vi "Fpga-Mac-Top.vi"(9 "RX_FIFO_DATA":refnum<k21>="TH-RX_FIFO_DATA", 10 "RX_PKT":refnum<k21>="TH-RX_NEW_PKT", 11 "TX_FIFO":refnum<k21>="HT-TX_FIFO") -> ()   [LabVIEW 2017]
uses:
  <instrlib>/_niInstr/Network/Ethernet/MAC/CLIP/v1/Resources.ctl
  TX-States.ctl
  <vilib>/Platform/TimedLoop/XDataNode/timing_clust.ctl
  <vilib>/Platform/TimedLoop/XDataNode/nitl_modes.ctl
  <vilib>/Platform/TimedLoop/XDataNode/wakeup.ctl
  <instrlib>/_niInstr/Network/Ethernet/MAC/Raw Stream/v1/niInstr Ethernet MAC Raw Stream v1.lvclass
  <instrlib>/_niInstr/Network/Ethernet/Utility/v1/FPGA/Network Data Stream.ctl
  <vilib>/rvi/Emulation/niFpgaSctlEmulationGetInTimedLoop.vi
  <vilib>/rvi/Emulation/niFpgaEmulationReportErrorSimple.vi
  <vilib>/rvi/Emulation/niFpgaGetClockAttributes.vi
  <vilib>/rvi/Emulation/niFpgaCriticalErrorInLSC.vi
  <vilib>/rvi/DataTransferAndStorage/Container/Common/niFpgaContainerExecOnDevCompGetState.vi
  <vilib>/rvi/Emulation/niFpgaEmulationIsFPGAContextNoSignature.vi
  <vilib>/rvi/errors/niFpgaSetErrorForExecOnDevCompSimple.vi
  <vilib>/rvi/eio/common/nirviEmuReportErrorAndStop.vi
  <vilib>/rvi/DataTransferAndStorage/Container/Common/niFpgaContainerGetUniqueNameForEmu.vi
  <vilib>/rvi/FIFO/Fifo_Resource/nirvififoEmulationSetSize.vi
  <vilib>/rvi/FIFO/Fifo_Resource/nirviFifoEmulationQueueMgr.vi
  <instcachedir>/0/nirviFifoEmulationQueueMgr_E5CAEC123FF24DC58D834DCA3CDAA9B5.lvgen/nirviFifoEmulationQueueMgr_E5CAEC123FF24DC58D834DCA3CDAA9B5_000.vi
  <vilib>/rvi/FIFO/Fifo_Resource/nirvififoEmulationDetermineInputValidOut.vi
  <vilib>/rvi/FIFO/Fifo_Resource/nirvififoEmulationCreateLock.vi
  <vilib>/rvi/Emulation/niFpgaProcessEmulError.vi
  <vilib>/rvi/FIFO/Fifo_Resource/nirvififoEmulationObtainLock.vi
  <vilib>/rvi/FIFO/Fifo_Resource/nirvififoEmulationReleaseLock.vi
  <vilib>/rvi/occurrence/nirviWaitOnOccurrenceBase.vi
  <vilib>/rvi/errors/nirviReportUnexpectedCaseInternalError.vi
  <vilib>/rvi/errors/nirviReportUnexpectedCaseInternalError (U32).vi
  <vilib>/Utility/error.llb/Clear Errors.vi
  <vilib>/rvi/interface/RandomDataEmulation/niFpgaRandomDataHandleErrors.vi
  <instrlib>/_niInstr/Network/Ethernet/MAC/Raw Stream/v1/Write Data Stream.vi
  <instrlib>/_niInstr/Network/Ethernet/MAC/Raw Stream/v1/Write End of Good Frame.vi
  <instrlib>/_niInstr/Network/Ethernet/MAC/Raw Stream/v1/Read End of Bad Frame.vi
  <instrlib>/_niInstr/Network/Ethernet/MAC/Raw Stream/v1/Read End of Good Frame.vi
  <instrlib>/_niInstr/Network/Ethernet/MAC/Raw Stream/v1/Read Data Stream.vi
  <vilib>/rvi/interface/RandomDataEmulation/nirviRandomDataAcquireLock.vi
  <vilib>/rvi/interface/RandomDataEmulation/nirviRandomDataQueueStore.vi
  <vilib>/rvi/interface/RandomDataEmulation/nirviRandomDataReleaseLock.vi
  <vilib>/rvi/interface/RandomDataEmulation/nirviFPGAContextMergeError.vi
  <vilib>/rvi/interface/RandomDataEmulation/nirviRandomDataCheckExitLoopConditions.vi
  <vilib>/express/rvi/timingcommon/nirviCommon.vi
  <instcachedir>/0/nirviFifoEmulationQueueMgr_E5CAEC123FF24DC58D834DCA3CDAA9B5.lvgen/nirviFifoEmulationQueueMgr_E5CAEC123FF24DC58D834DCA3CDAA9B5_007.vi
  <vilib>/rvi/eio/common/nirviEmuTemplateMethod_errors.vi
  <vilib>/Platform/TimedLoop/XDataNode/XDataNode.xnode
  <vilib>/rvi/DataTransferAndStorage/Container/XNode/niFpgaContainer.xnode
  <vilib>/rvi/FIFO/Fifo_Resource/niFpgaFifoEmulationRefIn.vi
  <vilib>/rvi/FIFO/Fifo_Resource/niFpgaFifoEmulationRefInMultiElement.vi
  <vilib>/eio/EIONode/EIONode.xnode
  <instrlib>/_niInstr/Network/Ethernet/MAC/CLIP/v1/niInstr Ethernet MAC - CLIP v1.lvclass
  <vilib>/Platform/TimedLoop/XDataNode/XDNodeRunTimeDep.lvlib
  <instrlib>/_niInstr/Network/Ethernet/Utility/v1/FPGA/niInstr Ethernet Utilities FPGA v1.lvlib
panel:
  out "mgtrefclks_locked":bool
  out "mgtrefclks_valid":bool
  out "posc_complete":bool
  out "sPort0_Power_Good":bool
  out "sPort1_Power_Good":bool
  out "signal_detect_Port0":bool
  out "signal_detect_Port1":bool
  out "aBlockLockPort0":bool
  out "aBlockLockPort1":bool
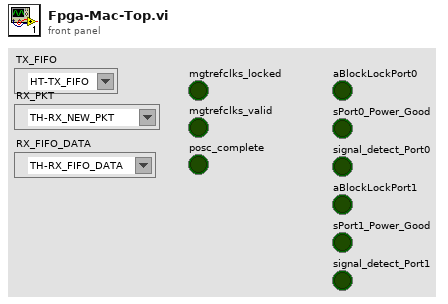
[diagram p1: front panel]
types:
  T1 = typedef "TX-States.ctl" = enum16{"Idle", "ReadSize", "WaitForData", "ReadData", "Reset", "InterFrameGap"}
  T2 = typedef "niInstr Ethernet MAC - CLIP v1.lvclass/Resources.ctl" = cluster{"RX":cluster{"TData":refnum<k21>, "TValid":refnum<k21>, "TKeep":refnum<k21>, "TLast":refnum<k21>, "TUser":refnum<k21>}, "TX":cluster{"TData":refnum<k21>, "TValid":refnum<k21>, "TKeep":refnum<k21>, "TLast":refnum<k21>, "TReady":refnum<k21>}, "Pause resources":cluster{"cPauseValuePort":refnum<k21>, "cPauseReqPort":refnum<k21>}, "MAC Clock":refnum<k21>}
  T3 = typedef "XDNodeRunTimeDep.lvlib/timing_clust.ctl" = cluster{"Expected End [f-1]":u64, "Actual End [f-1]":u64, "Finished Late? [f-1]":bool, "Expected End [i-1]":u64, "Actual End [i-1]":u64, "Finished Late? [i-1]":bool, "Expected Start [i]":u64, "Actual Start [i]":u64, "Expected Start [f]":u64, "Actual Start [f]":u64, "Source Name":string, "Structure Name":string, "Period":i64, "Deadline":i64, "Offset":i64, "Start":i64, "Priority":i32, "Timeout":i32, "Mode":T4, "Wakeup Reason":T5, "Error":errorcluster, "Source Type":string, "Secondary Source Type":string, "Global End Time":u64, "Global Start Time":u64, "Frame Duration":u64, "Iteration Duration":u64, "Assigned CPU":i32, "I/O Scan Engine Mode":u32}
  T4 = typedef "XDNodeRunTimeDep.lvlib/nitl_modes.ctl" = enum32{"No Change", "Process missed periods, maintain original phase", "Discard missed periods, maintain original phase", "Process missed periods, ignore original phase", "Discard missed periods, ignore original phase"}
  T5 = typedef "XDNodeRunTimeDep.lvlib/wakeup.ctl" = enum32{"Normal", "Aborted", "Asynchronous wakeup", "Timing source error", "Timed loop error", "Timeout"}
  T6 = cluster{"TotalBytes":u32, "TotalWords":u32, "Remainder":u32, "Counter":u32}
  T7 = typedef "niInstr Ethernet Utilities FPGA v1.lvlib/Network Data Stream.ctl" = cluster{"data":u8[], "data valid":bool, "byte enables":bool[]}
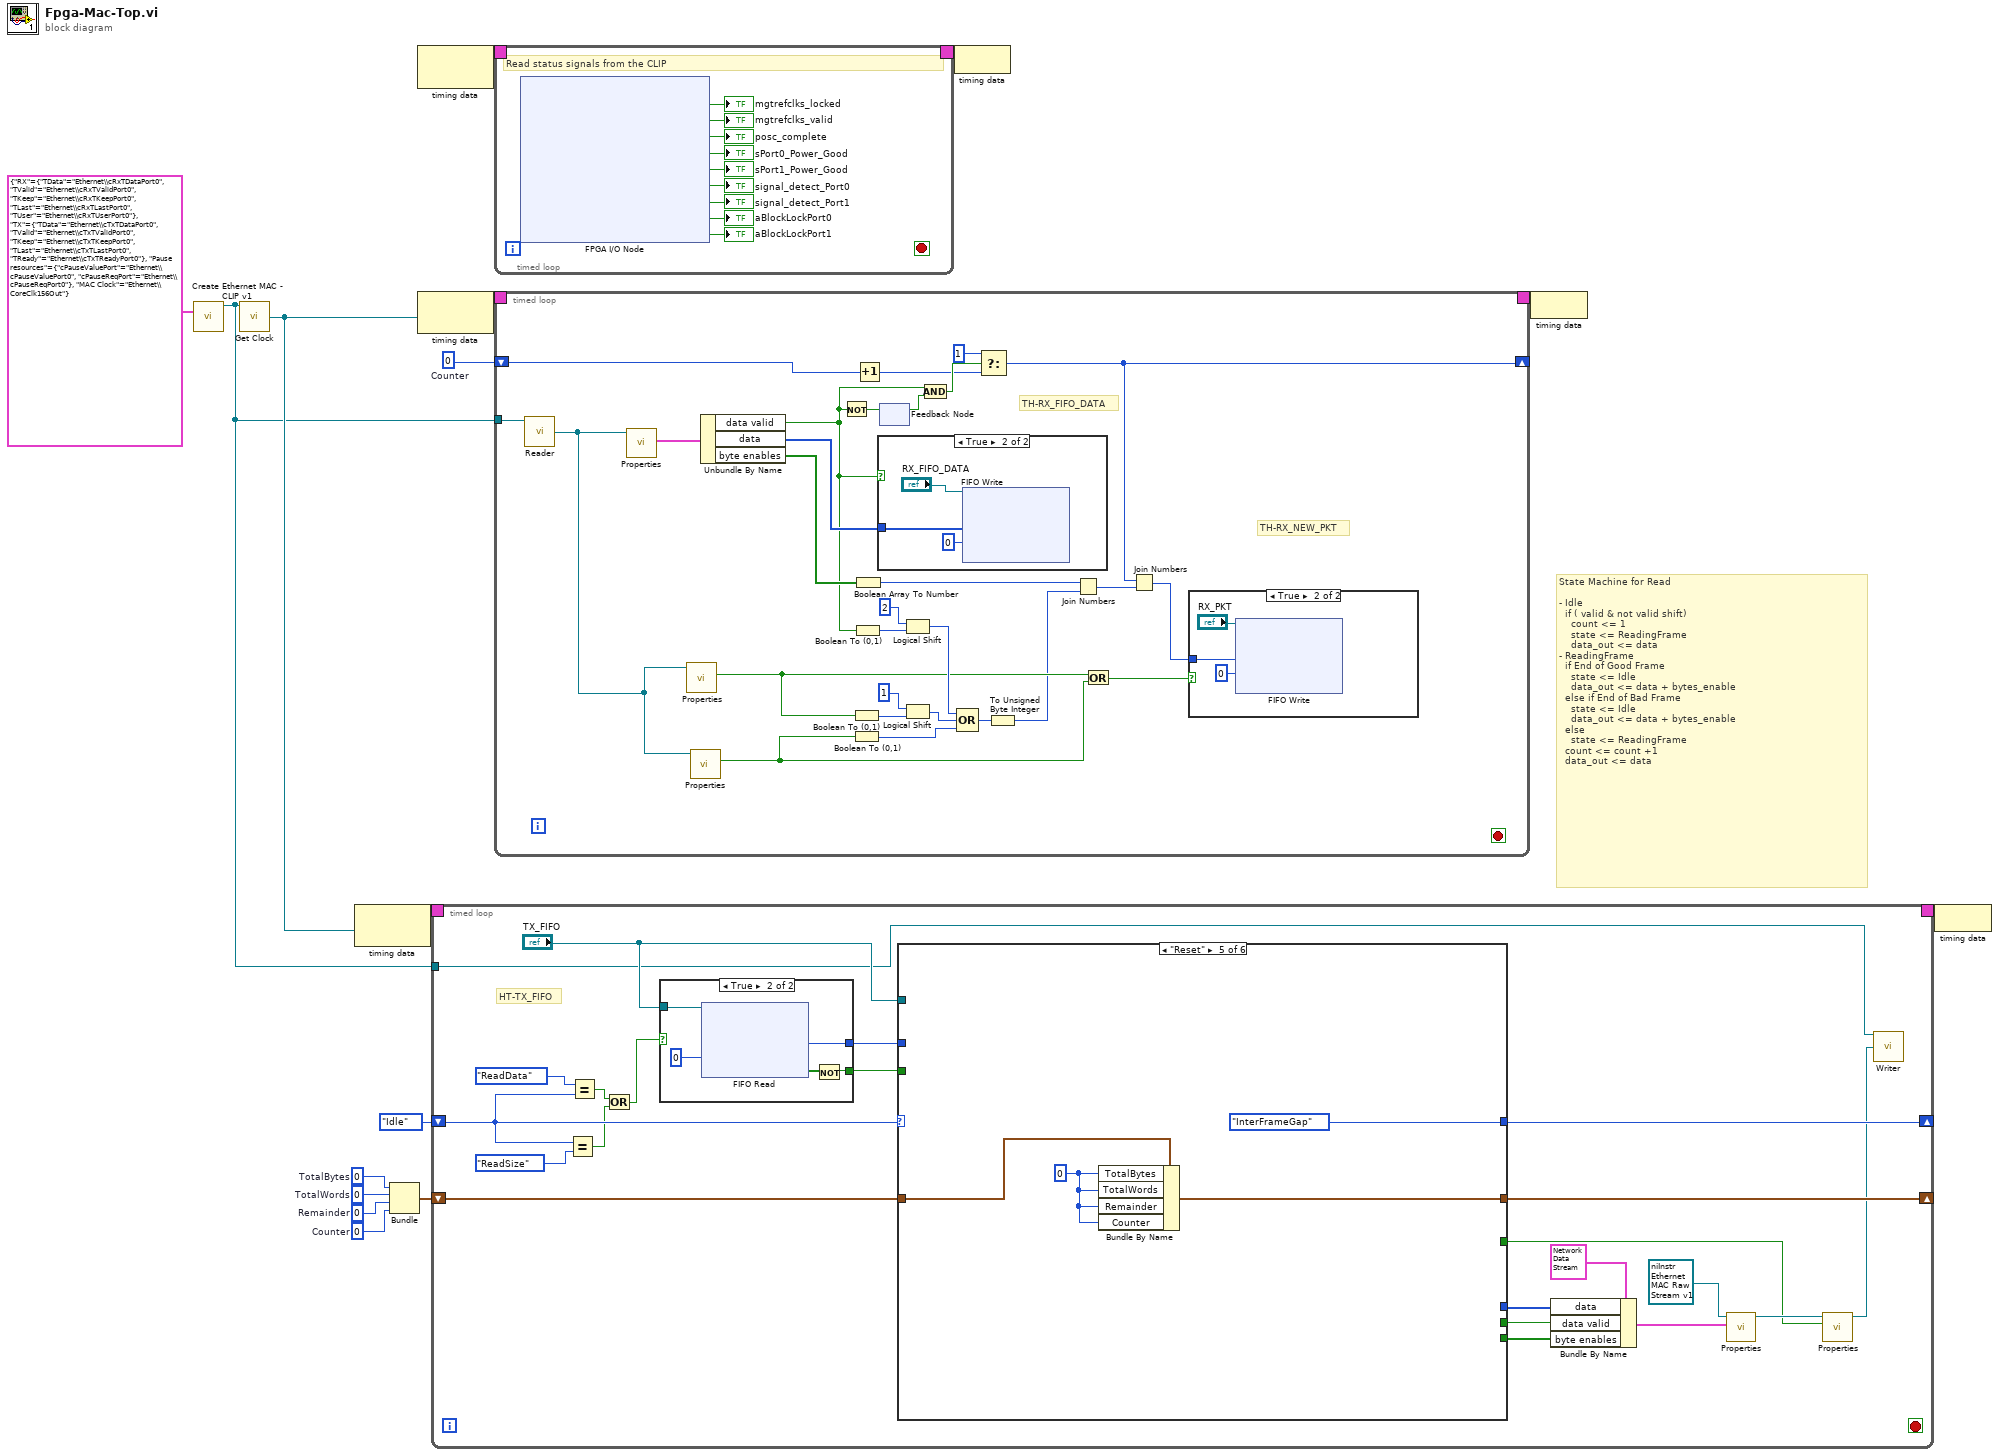
[diagram p0: block diagram]
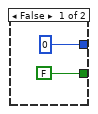
[diagram p2: hidden frame]
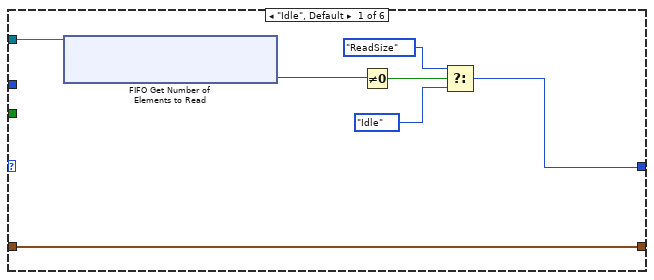
[diagram p3: hidden frame]
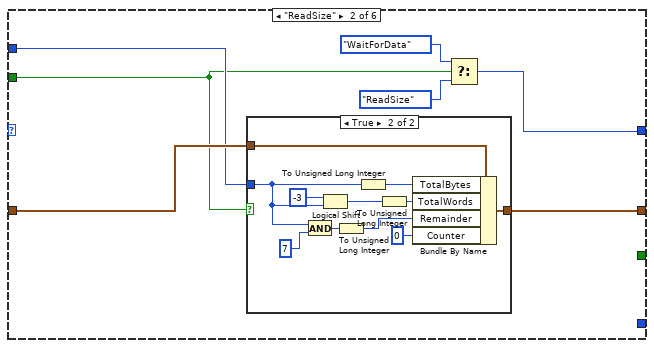
[diagram p4: hidden frame]
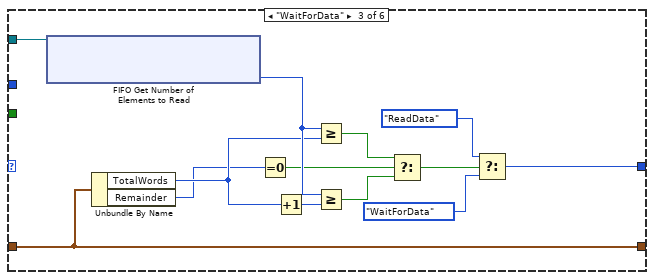
[diagram p6: hidden frame]
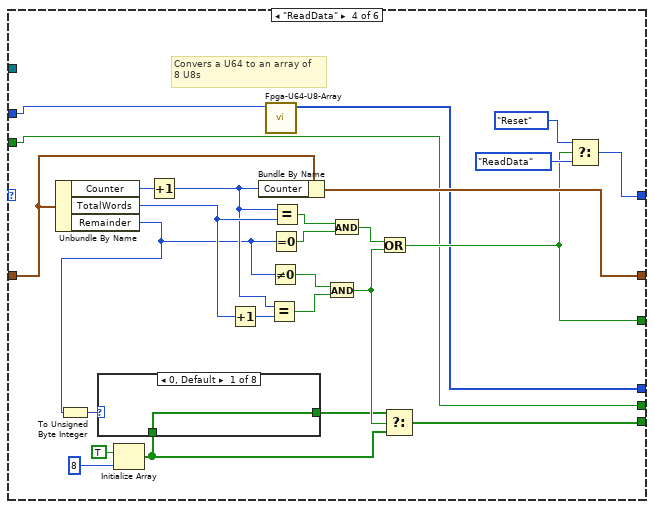
[diagram p7: hidden frame]
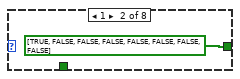
[diagram p8: hidden frame]
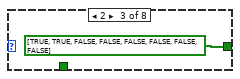
[diagram p9: hidden frame]
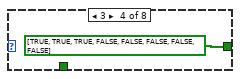
[diagram p10: hidden frame]
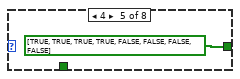
[diagram p11: hidden frame]
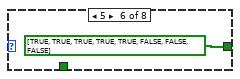
[diagram p12: hidden frame]
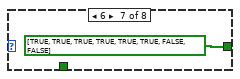
[diagram p13: hidden frame]
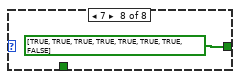
[diagram p14: hidden frame]
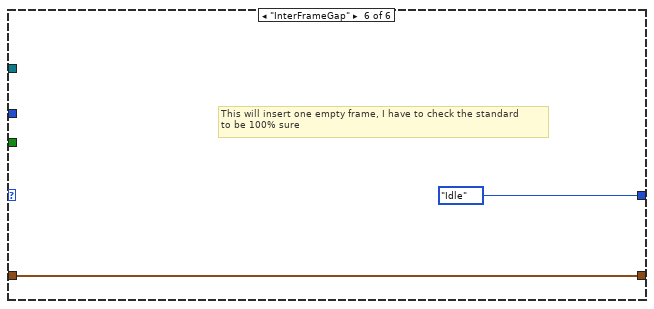
[diagram p15: hidden frame]
diagram:
  w1 = u16 0  # Counter
  w3 = u32 0  # Counter
  w4 = u32 0  # Remainder
  w5 = u32 0  # TotalWords
  w6 = u32 0  # TotalBytes
  # "State Machine for Read\n\n- Idle\n  if ( valid & not valid shift) \n    count <= 1\n    state <= ReadingFrame\n    data_out <= data\n- ReadingFrame\n  if End of Good Frame\n    state <= Idle\n    data_out <= data + bytes_enable\n  else if End of Bad Frame\n    state <= Idle\n    data_out <= data + bytes_enable\n  else\n    state <= ReadingFrame\n  count <= count +1\n  data_out <= data"
  n1 = call <instrlib>:"Create Ethernet MAC - CLIP v1.vi"("Ethernet AXI4-S Resources"=T2 {"RX"={"TData"="Ethernet\\cRxTDataPort0", "TValid"="Ethernet\\cRxTValidPort0", "TKeep"="Ethernet\\cRxTKeepPort0", "TLast"="Ethernet\\cRxTLastPort0", "TUser"="Ethernet\\cRxTUserPort0"}, "TX"={"TData"="Ethernet\\cTxTDataPort0", "TValid"="Ethernet\\cTxTValidPort0", "TKeep"="Ethernet\\cTxTKeepPort0", "TLast"="Ethernet\\cTxTLastPort0", "TReady"="Ethernet\\cTxTReadyPort0"}, "Pause resources"={"cPauseValuePort"="Ethernet\\cPauseValuePort0", "cPauseReqPort"="Ethernet\\cPauseReqPort0"}, "MAC Clock"="Ethernet\\CoreClk156Out"}) -> ("niInstr Ethernet MAC - CLIP v1.lvclass out"=w8:refnum<class "niInstr Ethernet MAC - CLIP v1.lvclass">)  [unwired: 14 in]
  n2 = call-dynamic "Get Clock.vi"("niInstr Ethernet MAC - CLIP v1.lvclass"=w8) -> ("MAC Clock"=w9:refnum<k21>)  [unwired: 14 in]
  n3 = node-c288(w9) -> (w11:T3)
  n4 = Bundle("TotalBytes"=w6, "TotalWords"=w5, "Remainder"=w4, "Counter"=w3) -> (w2:T6)  [unwired: 1 in]
  n5 = node-c288() -> (w14:T3)  [unwired: 1 in]
  n6 = node-c288(w9) -> (w16:T3)
  n7 = timed-loop {
    timing: w11 -> [_]
    timing-out: [_] -> w10
    tunnel: w8 -> [w26]
    shift-right: [w38] -> _
    shift-left: TX-States."Idle" -> [w31]
    shift-right: [w36] -> _
    shift-left: w2 -> [w37]
    stop <- _ stop-if-true
    # "HT-TX_FIFO"
    n8 = Equal?(x=w31, y=TX-States."ReadSize") -> (x = y?=w29:bool)
    n9 = Equal?(x=TX-States."ReadData", y=w31) -> (x = y?=w28:bool)
    n10 = Or(x=w28, y=w29) -> (x .or. y?=w27:bool)
    n11 = case shown="True" w27 {
      tunnel: "TX_FIFO" -> [_ w44]
      tunnel: [u64 0 ("Element") w42] -> w35
      tunnel: [FALSE w41] -> w34
      frame False {
      }
      frame True {
        n12 = xnode ("FIFO Read")("Timeout"=0, "FIFO In"=w44) -> ("Element"=w42:u64, "Timed Out?"=w43:bool)  [unwired: 1 out]
        n13 = Not(x=w43) -> (.not. x?=w41:bool)
      }
    }
    n14 = case shown="\"Reset\"" w31 {
      tunnel: [w49 w55 w77 w108 TX-States."InterFrameGap" TX-States."Idle"] -> w38
      tunnel: w37 -> [w48 w59 w73 w106 w120 w124]
      tunnel: [w48 w58 w73 w105 w121 w124] -> w36
      tunnel: w34 -> [_ w53 _ w86 _ _]
      tunnel: w35 -> [_ w54 _ w95 _ _]
      tunnel: "TX_FIFO" -> [w47 _ w72 _ _ _]
      tunnel: [_ _ _ w88 _ _] -> w22
      tunnel: [_ _ _ w87 _ _] -> w21
      tunnel: [_ _ _ w86 _ _] -> w20
      tunnel: [_ _ _ w85 _ _] -> w19
      frame "Idle", Default {
        n15 = xnode ("FIFO Get Number of Elements to Read")("FIFO In"=w47) -> ("Number of Elements to Read"=w46:u32)  [unwired: 1 out]
        n16 = Not Equal To 0?(x=w46) -> (x != 0?=w52:bool)
        n17 = Select(t=TX-States."ReadSize", s=w52, f=TX-States."Idle") -> (s? t:f=w49:T1)
      }
      frame "ReadSize" {
        n18 = case shown="True" w53 {
          tunnel: w59 -> [w60 w71]
          tunnel: [w60 w70] -> w58
          tunnel: w54 -> [_ w61]
          frame False {
          }
          frame True {
            n19 = And(x=w61, y=u64 7) -> (x .and. y?=w63:u64)
            n20 = Logical Shift(y=i16 -3, x=w61) -> (x << y=w66:u64)
            n21 = To Unsigned Long Integer(number=w63) -> (unsigned 32bit integer=w64:u32)
            n22 = To Unsigned Long Integer(number=w61) -> (unsigned 32bit integer=w69:u32)
            n23 = To Unsigned Long Integer(number=w66) -> (unsigned 32bit integer=w65:u32)
            n24 = Bundle By Name(cluster=w71, "TotalBytes"=w69, "TotalWords"=w65, "Remainder"=w64, "Counter"=u32 0) -> (w70:T6)
          }
        }
        n25 = Select(t=TX-States."WaitForData", s=w53, f=TX-States."ReadSize") -> (s? t:f=w55:T1)
      }
      frame "WaitForData" {
        n26 = xnode ("FIFO Get Number of Elements to Read")("FIFO In"=w72) -> ("Number of Elements to Read"=w84:u32)  [unwired: 1 out]
        n27 = Unbundle By Name(w73) -> ("TotalWords"=w83:u32, "Remainder"=w81:u32)
        n28 = Equal To 0?(x=w81) -> (x = 0?=w78:bool)
        n29 = Increment(x=w83) -> (x+1=w82:u32)
        n30 = Greater Or Equal?(x=w84, y=w83) -> (x >= y?=w80:bool)
        n31 = Greater Or Equal?(x=w84, y=w82) -> (x >= y?=w79:bool)
        n32 = Select(t=w80, s=w78, f=w79) -> (s? t:f=w74:bool)
        n33 = Select(t=TX-States."ReadData", s=w74, f=TX-States."WaitForData") -> (s? t:f=w77:T1)
      }
      frame "ReadData" {
        # "Convers a U64 to an array of \n8 U8s"
        n34 = Unbundle By Name(w106) -> ("Counter"=w107:u32, "TotalWords"=w98:u32, "Remainder"=w96:u32)
        n35 = To Unsigned Byte Integer(number=w96) -> (unsigned 8bit integer=w94:u8)
        n36 = Initialize Array(TRUE, i8 8 ("y")) -> (w89:bool[])
        n37 = case shown="0, Default" w94 {
          tunnel: [w111 bool[] [TRUE, FALSE, FALSE, FALSE, FALSE, FALSE, FALSE, FALSE] bool[] [TRUE, TRUE, FALSE, FALSE, FALSE, FALSE, FALSE, FALSE] bool[] [TRUE, TRUE, TRUE, FALSE, FALSE, FALSE, FALSE, FALSE] bool[] [TRUE, TRUE, TRUE, TRUE, FALSE, FALSE, FALSE, FALSE] bool[] [TRUE, TRUE, TRUE, TRUE, TRUE, FALSE, FALSE, FALSE] bool[] [TRUE, TRUE, TRUE, TRUE, TRUE, TRUE, FALSE, FALSE] bool[] [TRUE, TRUE, TRUE, TRUE, TRUE, TRUE, TRUE, FALSE]] -> w90
          tunnel: w89 -> [w111 _ _ _ _ _ _ _]
          frame 0, Default {
          }
          frame 1 {
          }
          frame 2 {
          }
          frame 3 {
          }
          frame 4 {
          }
          frame 5 {
          }
          frame 6 {
          }
          frame 7 {
          }
        }
        n38 = Increment(x=w107) -> (x+1=w97:u32)
        n39 = Increment(x=w98) -> (x+1=w99:u32)
        n40 = Bundle By Name(cluster=w106, "Counter"=w97) -> (w105:T6)
        n41 = call "Fpga-U64-U8-Array.vi"("U64 in"=w95) -> ("U8[] out"=w87:u8[])  [unwired: 10 in]
        n42 = Equal?(x=w97, y=w99) -> (x = y?=w100:bool)
        n43 = Not Equal To 0?(x=w96) -> (x != 0?=w101:bool)
        n44 = Equal To 0?(x=w96) -> (x = 0?=w103:bool)
        n45 = Equal?(x=w97, y=w98) -> (x = y?=w104:bool)
        n46 = And(x=w101, y=w100) -> (x .and. y?=w91:bool)
        n47 = And(x=w104, y=w103) -> (x .and. y?=w102:bool)
        n48 = Or(x=w102, y=w91) -> (x .or. y?=w88:bool)
        n49 = Select(t=w90, s=w91, f=w89) -> (s? t:f=w85:bool[])
        n50 = Select(t=TX-States."Reset", s=w88, f=TX-States."ReadData") -> (s? t:f=w108:T1)
      }
      frame "Reset" {
        w119 = u32 0 ("TotalBytes")
        n51 = Bundle By Name(cluster=w120, "TotalBytes"=w119, "TotalWords"=w119, "Remainder"=w119, "Counter"=w119) -> (w121:T6)
      }
      frame "InterFrameGap" {
        # "This will insert one empty frame, I have to check the standard \nto be 100% sure"
      }
    }
    n52 = Bundle By Name(cluster=T7 {"data"=[0, 0, 0, 0, 0, 0, 0, 0], "data valid"=FALSE, "byte enables"=[FALSE, FALSE, FALSE, FALSE, FALSE, FALSE, FALSE, FALSE]} ("Data Stream"), "data"=w21, "data valid"=w20, "byte enables"=w19) -> (w24:T7)
    n53 = call-poly <instrlib>:"Properties.vi"("Data Stream"=w24, "niInstr Ethernet MAC Data Stream v1 in"=refnum<class "niInstr Ethernet MAC Raw Stream v1.lvclass"> refnum) -> ("niInstr Ethernet MAC Data Stream v1 out"=w23:refnum<class "niInstr Ethernet MAC Raw Stream v1.lvclass">)  [unwired: 9 in]
    n54 = call-poly <instrlib>:"Properties.vi"("End of Good Frame"=w22, "niInstr Ethernet MAC Data Stream v1 in"=w23) -> ("niInstr Ethernet MAC Data Stream v1 out"=w17:refnum<class "niInstr Ethernet MAC Raw Stream v1.lvclass">)  [unwired: 9 in]
    n55 = call-dynamic "Writer.vi"("niInstr Ethernet MAC v1.lvclass"=w26, "niInstr Ethernet MAC Raw Stream v1.lvclass"=w17) -> ()  [unwired: 12 in, 2 out]
  }
  n56 = timed-loop {
    timing: w14 -> [_]
    timing-out: [_] -> w13
    stop <- _ stop-if-true
    # "Read status signals from the CLIP"
    n57 = xnode "FPGA I/O Node"() -> ("Ethernet\\MgtRefClks_Locked"=→"mgtrefclks_locked":bool, "Ethernet\\MgtRefClks_Valid"=→"mgtrefclks_valid":bool, "Ethernet\\POSC_Complete"=→"posc_complete":bool, "Ethernet\\sPort0_Power_Good"=→"sPort0_Power_Good":bool, "Ethernet\\sPort1_Power_Good"=→"sPort1_Power_Good":bool, "Ethernet\\signal_detect_Port0"=→"signal_detect_Port0":bool, "Ethernet\\signal_detect_Port1"=→"signal_detect_Port1":bool, "Ethernet\\aBlockLockPort0"=→"aBlockLockPort0":bool, "Ethernet\\aBlockLockPort1"=→"aBlockLockPort1":bool)  [unwired: 9 in, 9 out]
  }
  n58 = timed-loop {
    timing: w16 -> [_]
    timing-out: [_] -> w15
    tunnel: w8 -> [w165]
    shift-right: [w154] -> _
    shift-left: w1 -> [w160]
    stop <- _ stop-if-true
    # "TH-RX_NEW_PKT"
    # "TH-RX_FIFO_DATA"
    n59 = call-dynamic "Reader.vi"("niInstr Ethernet MAC - CLIP v1.lvclass 2"=w165) -> ("niInstr Ethernet MAC Raw Stream v1.lvclass"=w156:refnum<class "niInstr Ethernet MAC Raw Stream v1.lvclass">)  [unwired: 13 in, 1 out]
    n60 = call-poly <instrlib>:"Properties.vi"("niInstr Ethernet MAC Data Stream v1 in"=w156) -> ("Data Stream"=w164:T7)  [unwired: 9 in, 1 out]
    n61 = call-poly <instrlib>:"Properties.vi"("niInstr Ethernet MAC Data Stream v1 in"=w156) -> ("End of Good Frame"=w141:bool)  [unwired: 9 in, 1 out]
    n62 = call-poly <instrlib>:"Properties.vi"("niInstr Ethernet MAC Data Stream v1 in"=w156) -> ("End of Bad Frame"=w140:bool)  [unwired: 9 in, 1 out]
    n63 = Unbundle By Name(w164) -> ("data valid"=w142:bool, "data"=w157:u8[], "byte enables"=w155:bool[])
    n64 = Not(x=w142) -> (.not. x?=w163:bool)
    n65 = Boolean To (0,1)(Boolean=w141) -> (0, 1=w150:i16)
    n66 = Boolean To (0,1)(Boolean=w140) -> (0, 1=w148:i16)
    n67 = Boolean To (0,1)(Boolean=w142) -> (0, 1=w146:i16)
    n68 = Boolean Array To Number(Boolean array=w155) -> (number=w143:u8)
    n69 = Increment(x=w160) -> (x+1=w159:u16)
    n70 = case shown="True" w142 {
      tunnel: w157 -> [_ w171]
      frame False {
      }
      frame True {
        n71 = xnode ("FIFO Write")("Element"=w171, "Timeout"=0, "FIFO In"="RX_FIFO_DATA") -> ()  [unwired: 2 out]
      }
    }
    n72 = feedback-in #1(w163) -> ()
    n73 = feedback #1() -> (w162:bool)  [unwired: 1 in]
    n74 = Logical Shift(y=i16 2, x=w146) -> (x << y=w144:i16)
    n75 = Logical Shift(y=i16 1, x=w150) -> (x << y=w149:i16)
    n76 = And(x=w142, y=w162) -> (x .and. y?=w161:bool)
    n77 = Compound Arithmetic op=OR(w144, w149, w148) -> (w151:i16)
    n78 = Select(t=u16 1, s=w161, f=w159) -> (s? t:f=w154:u16)
    n79 = To Unsigned Byte Integer(number=w151) -> (unsigned 8bit integer=w138:u8)
    n80 = Join Numbers(hi=w143, lo=w138) -> ((hi.lo)=w152:u16)
    n81 = Or(x=w141, y=w140) -> (x .or. y?=w139:bool)
    n82 = Join Numbers(hi=w154, lo=w152) -> ((hi.lo)=w153:u32)
    n83 = case shown="True" w139 {
      tunnel: w153 -> [_ w168]
      frame False {
      }
      frame True {
        n84 = xnode ("FIFO Write")("Element"=w168, "Timeout"=0, "FIFO In"="RX_PKT") -> ()  [unwired: 2 out]
      }
    }
  }
  n85 = node-c288(w13) -> ()
  n86 = node-c288(w15) -> ()
  n87 = node-c288(w10) -> ()
